vi "Configure daqmx.vi"(8 "error in (no error)":errorcluster, 11 "measurement configuration":T1 {"PAYLOAD" format="%x"; "IDENTIFIER" format="%x"; "Baudrate" format="%x"; "FD Baudrate" format="%x"; "Active Edge" items=["Rising"=10280, "Falling"=10171]}) -> (0 "error out":errorcluster, 2 "Pulses":u32, 3 "Task out":refnum<k21>, 5 "Timeout":dbl)   [LabVIEW 2025, in "Workflow DO.lvclass"]
uses:
  Workflow DO.lvclass
  Measurement Configuration.ctl
  <vilib>/DAQmx/create/channels.llb/DAQmx Create Channel (CI-Count Edges).vi
  Workflow DO.lvclass/Workflow DO.ctl
  <resource>/objmgr/daqmx.rc
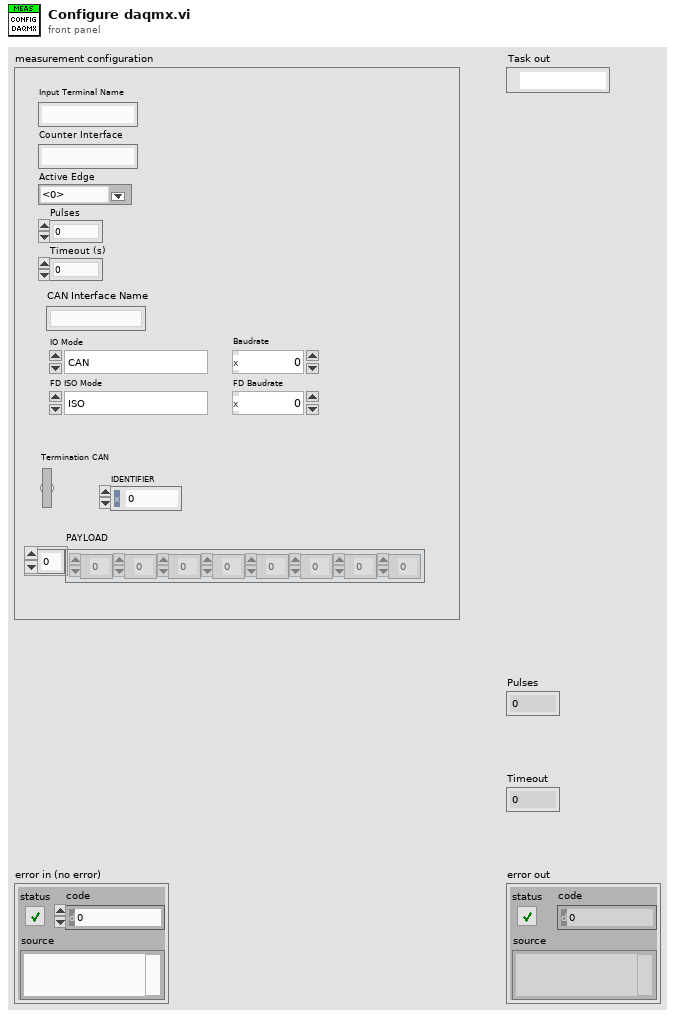
[diagram p1: front panel]
types:
  T1 = typedef "Workflow DO.lvclass/Measurement Configuration.ctl" = cluster{"Input Terminal Name":string, "Counter Interface":string, "Active Edge":i32, "Pulses":u32, "Timeout (s)":u32, "FD Baudrate":u32, "Baudrate":u32, "FD ISO Mode":enum32{"ISO", "Legacy ISO", "Non-ISO"}, "IO Mode":enum32{"CAN", "CAN FD", "CAN FD + BRS"}, "CAN Interface Name":string, "Termination CAN":bool, "IDENTIFIER":u32, "PAYLOAD":u32[]}
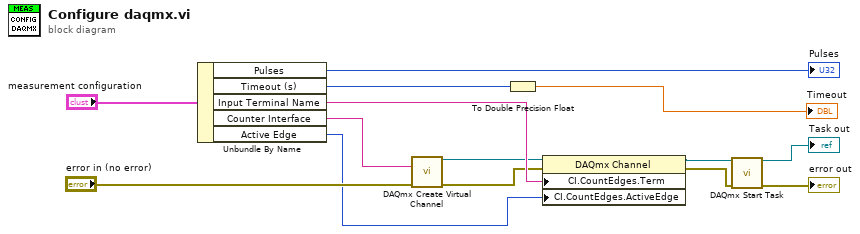
[diagram p0: block diagram]
diagram:
  n1 = Unbundle By Name("measurement configuration") -> ("Pulses"=→"Pulses":u32, "Timeout (s)"=w11:u32, "Input Terminal Name"=w4:string, "Counter Interface"=w5:string, "Active Edge"=w6:i32)
  n2 = call-poly <vilib>:"DAQmx Create Virtual Channel.vi"("counter"=w5, "error in"="error in (no error)") -> ("task out"=w1:refnum<k21>, "error out"=w2:errorcluster)  [unwired: 12 in]
  n3 = To Double Precision Float(number=w11) -> (double precision float=→"Timeout":dbl)
  n4 = property class="DAQmx Channel"(reference=w1, error in=w2, "CI.CountEdges.Term"=w4, "CI.CountEdges.ActiveEdge"=w6) -> (reference out=w7:refnum<k21>, error out=w9:errorcluster)
  n5 = call <vilib>:"DAQmx Start Task.vi"("task/channels in"=w7, "error in"=w9) -> ("task out"=→"Task out":refnum<k21>, "error out"=→"error out":errorcluster)  [unwired: 12 in]
